vi "Read Value.vi"(8 "error in (no error)":errorcluster, 11 "Double Parameter in":refnum<class "Double Parameter.lvclass">) -> (0 "error out":errorcluster, 2 "Value":dbl, 3 "Double Parameter out":refnum<class "Double Parameter.lvclass">)   [LabVIEW 2019, in "CD Parameter Manager API.lvlib" / "Double Parameter.lvclass"]
uses:
  Double Parameter.lvclass
  Double Parameter.lvclass/Double Parameter.ctl
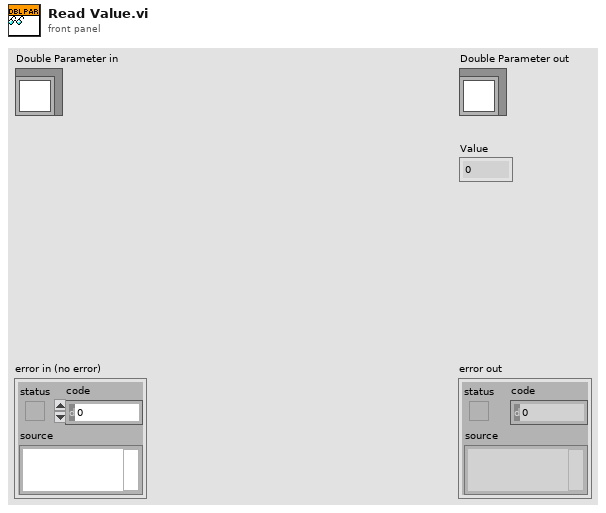
[diagram p1: front panel]
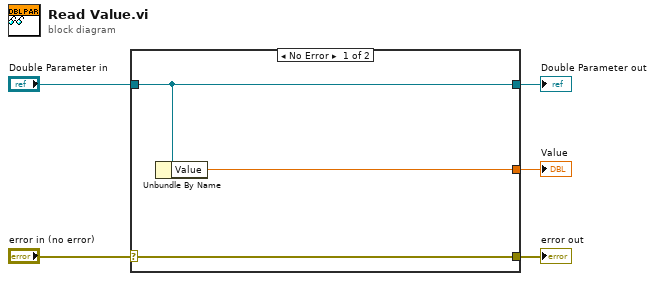
[diagram p0: block diagram]
diagram:
  n1 = case shown="No Error" "error in (no error)" {
    selector: "error in (no error)" -> [w8 w9]
    tunnel: [w8 w9] -> w4
    tunnel: [w7 w10] -> w2
    tunnel: "Double Parameter in" -> [w7 w10]
    tunnel: [w6 _] -> w1
    frame No Error {
      n2 = Unbundle By Name(w7) -> ("Value"=w6:dbl)
    }
    frame Error {
    }
  }
  "error out" <- w4
  "Double Parameter out" <- w2
  "Value" <- w1
